vi "DDSBox.vi"() -> ()   [LabVIEW 2014]
uses:
  <vilib>/Utility/file.llb/Write To Spreadsheet File (DBL).vi
  <vilib>/Utility/file.llb/Read From Spreadsheet File (DBL).vi
panel:
  in  "Reset":bool=TRUE
  in  "stop":bool
  in  "Save":bool
  in  "Profile File":path=path "D:/app/DDS/DDSBox/DDSBox.csv"
  in  "Channel":u32(ring) items=["0", "1", "2", "3"]
  in  "Profiles":T1(array[cluster]) {"Phase (Pi)" min=0.0 max=2.0 format="%.2f"; "Amplitude" min=0.0 max=1.0 format="%.2f"; "Frequency (MHz)" min=0.0 max=500.0 format="%.6f"}
  in  "Port":refnum<visa-resource-name>="COM16"
  in  "Profile":u32(ring) items=["0", "1", "2", "3", "4", "5", "6", "7"]
  in  "Phase (Pi)":dbl min=0.0 max=2.0 format="%.2f"
  in  "Frequency (MHz)":dbl=200.0 min=0.0 max=500.0 format="%.6f"
  in  "Amplitude":dbl=1.0 min=0.0 max=1.0 format="%.2f"
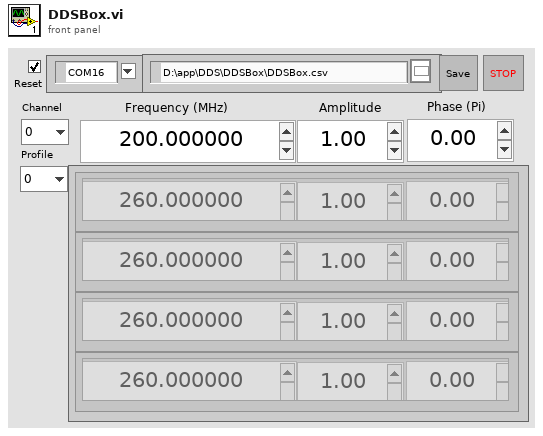
[diagram p1: front panel]
types:
  T1 = cluster{"Frequency (MHz) ":dbl, "Amplitude ":dbl, "Phase (Pi) ":dbl}[][]
  T2 = cluster{"Frequency (MHz) ":dbl, "Amplitude ":dbl, "Phase (Pi) ":dbl}
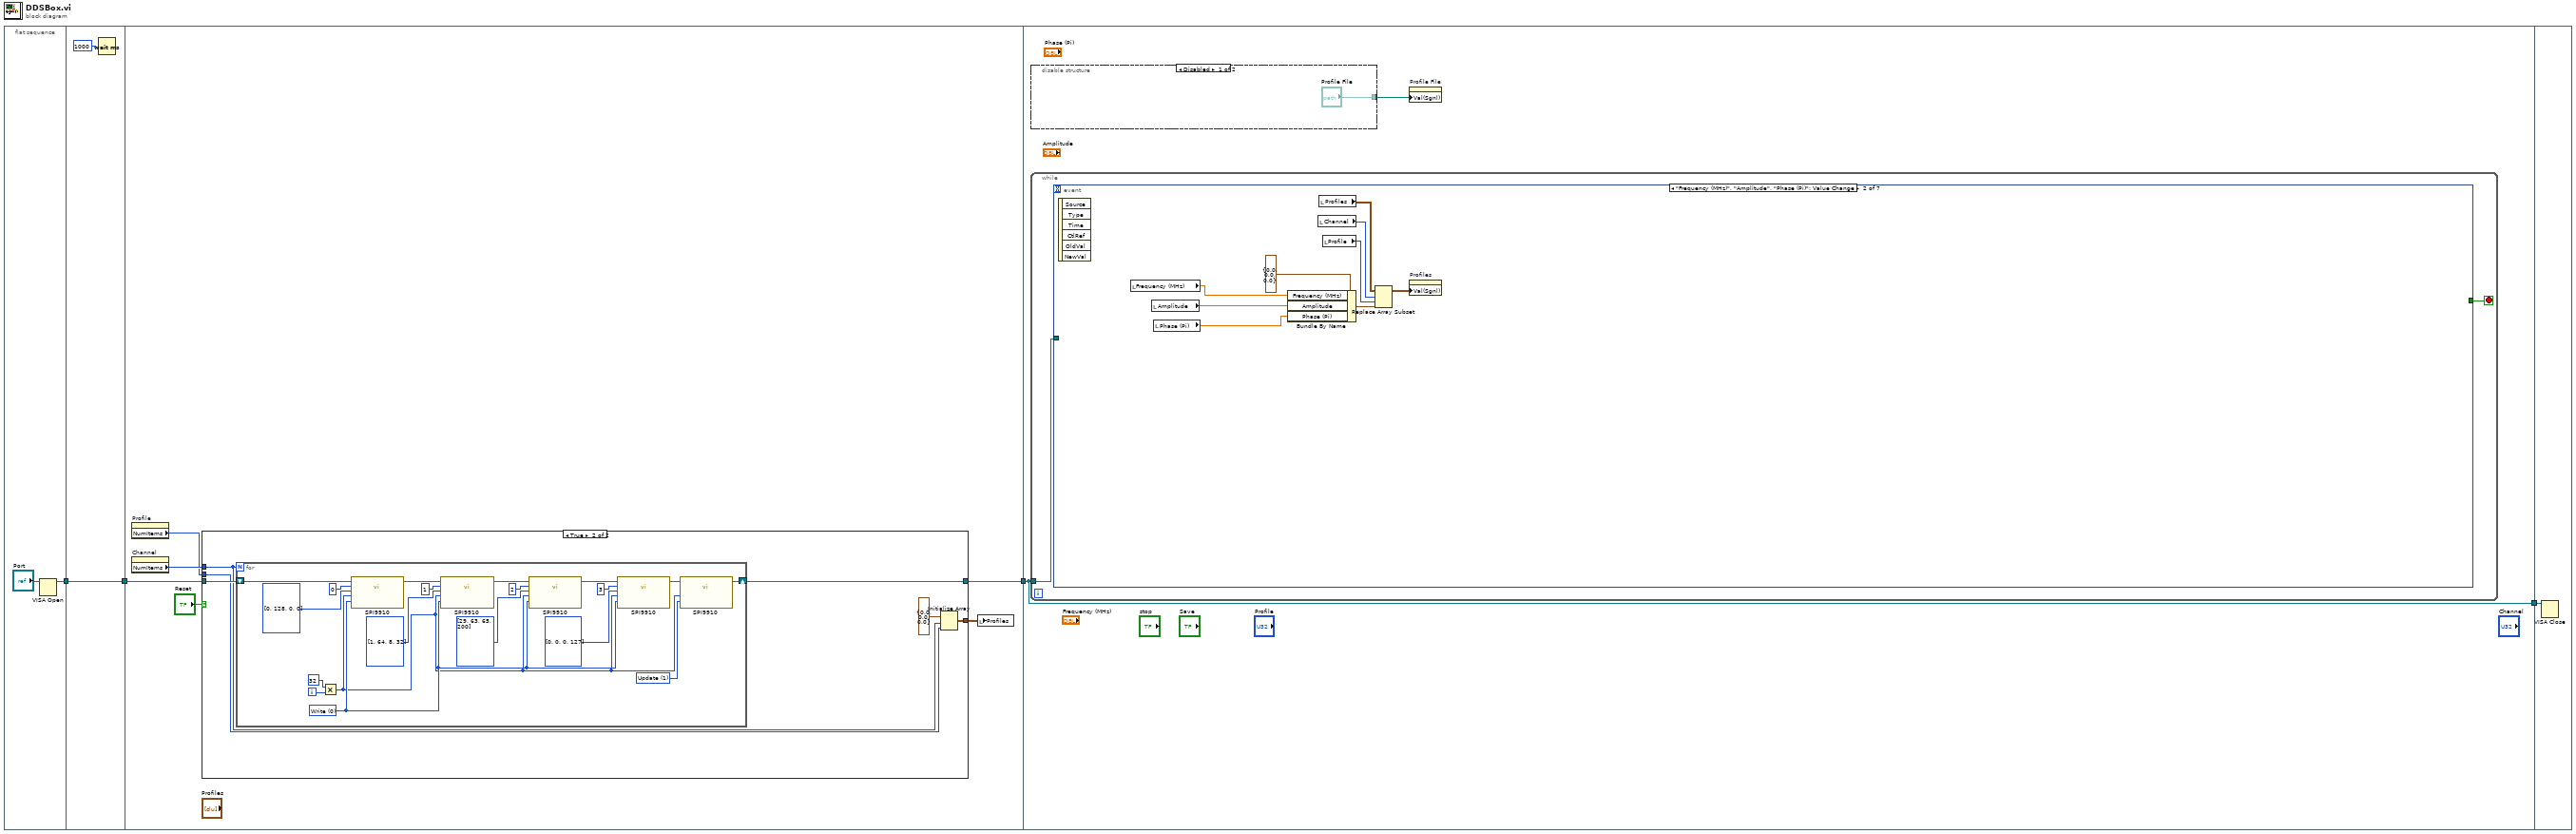
[diagram p0: block diagram]
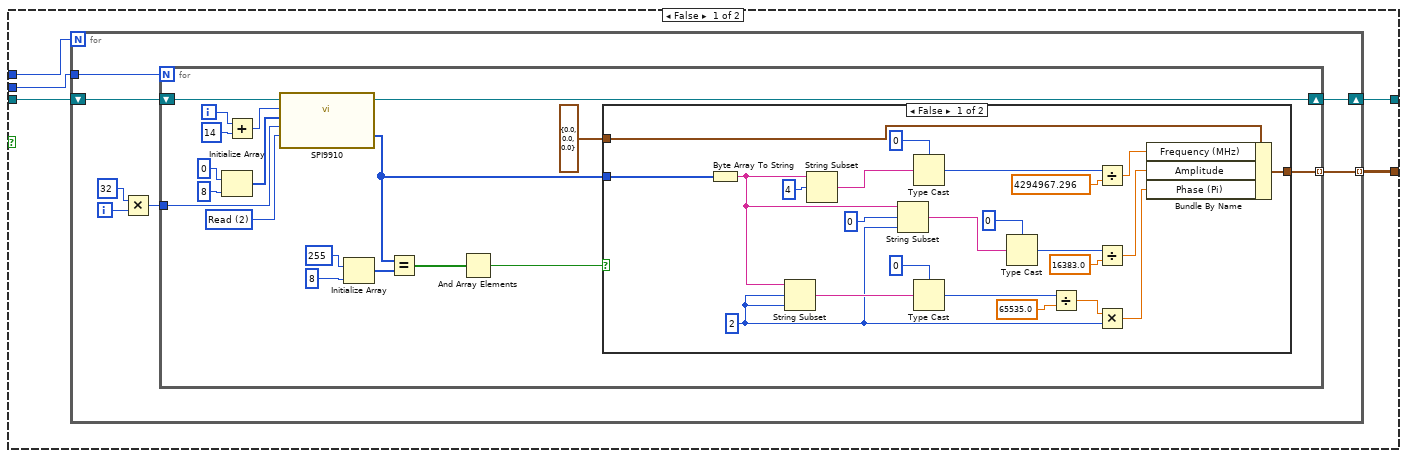
[diagram p2: hidden frame]
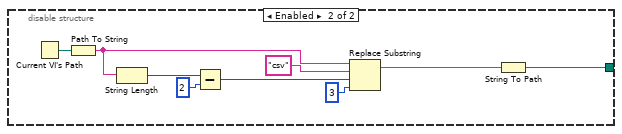
[diagram p4: hidden frame]
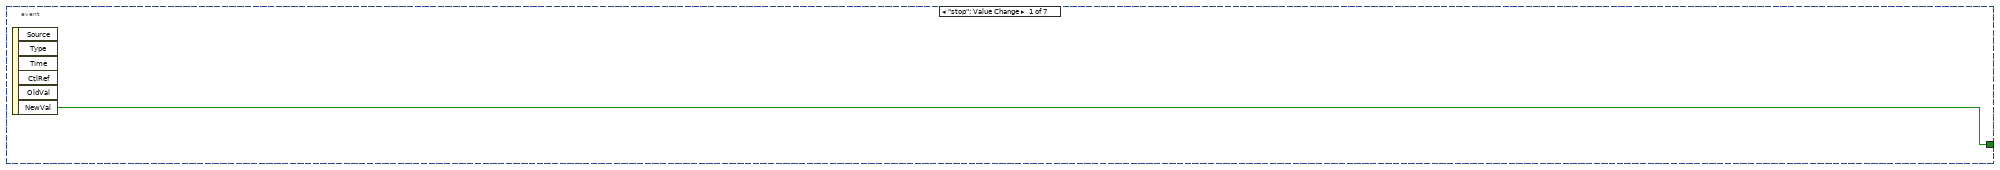
[diagram p5: hidden frame]
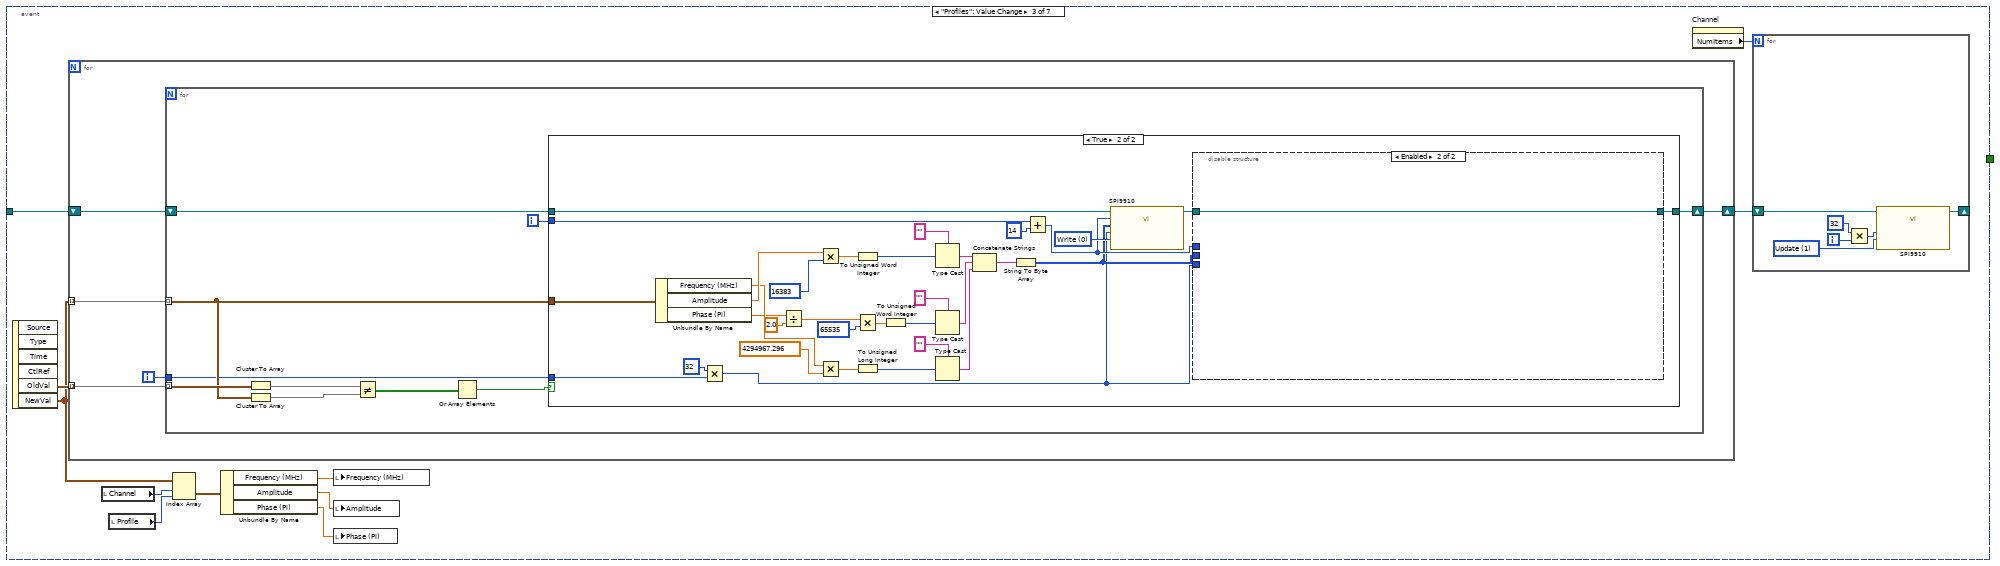
[diagram p6: hidden frame]
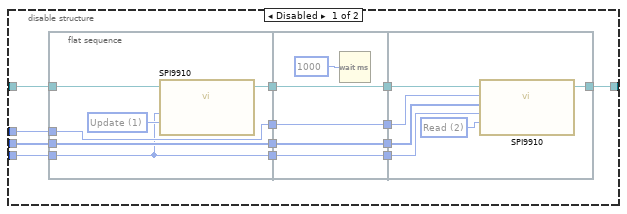
[diagram p8: hidden frame]
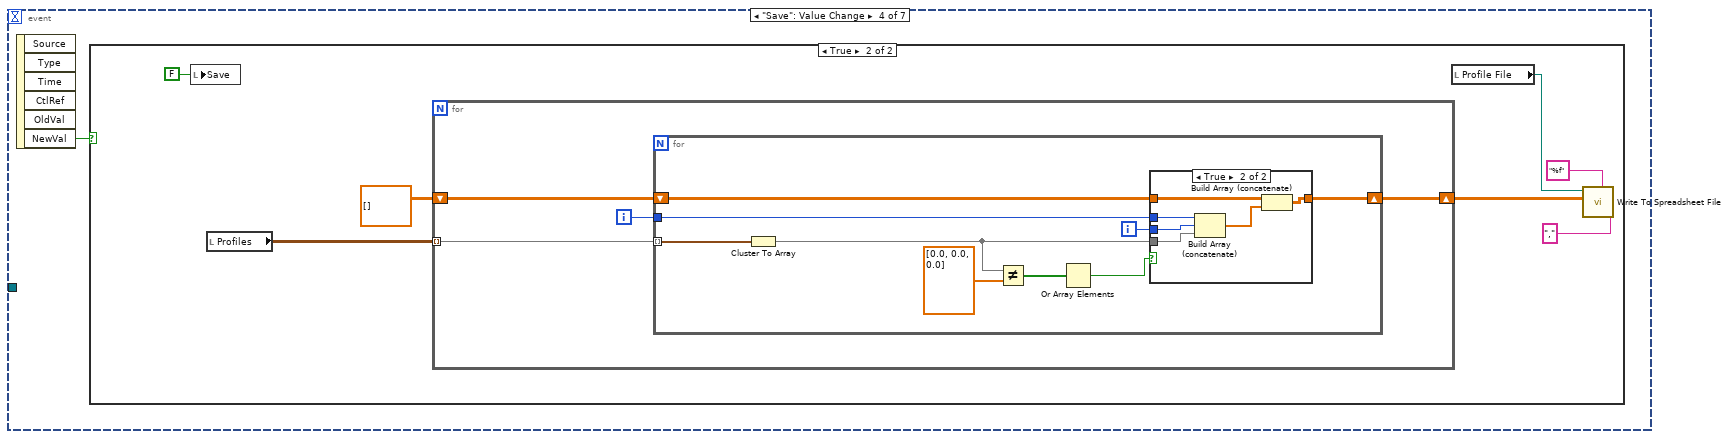
[diagram p9: hidden frame]
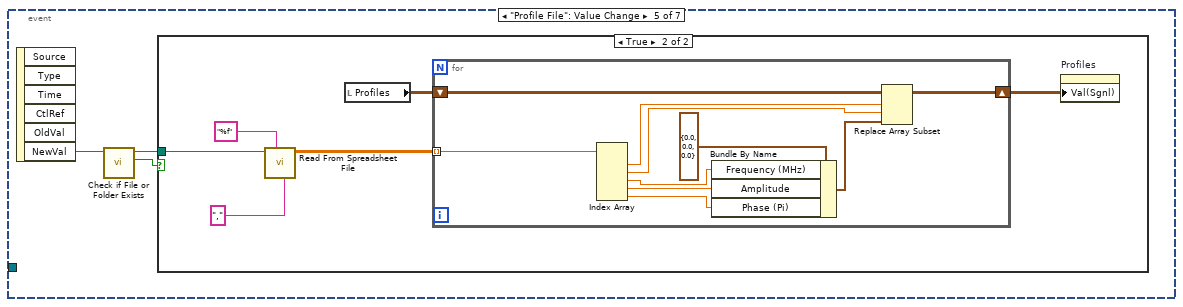
[diagram p12: hidden frame]
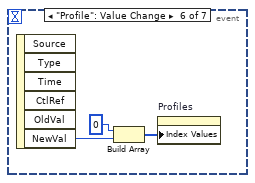
[diagram p14: hidden frame]
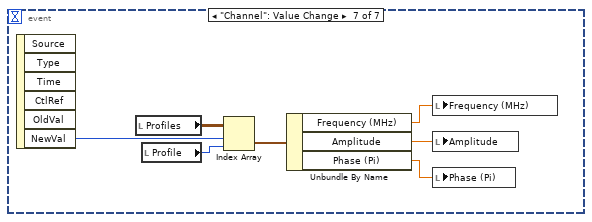
[diagram p15: hidden frame]
diagram:
  n1 = flat-sequence {
    tunnel: [w5] -> w2
    tunnel: w2 -> [w7]
    tunnel: [w7] -> w1
    tunnel: [w14] -> w3
    tunnel: w1 -> [w13]
    tunnel: w3 -> [w95]
    tunnel: [w95] -> w4
    tunnel: w4 -> [w272]
    frame #0 {
      n2 = VISA Open(VISA resource name="Port") -> (VISA resource name=w5:refnum<visa-resource-name>)  [unwired: 4 in, 1 out]
    }
    frame #1 {
      n3 = Wait (ms)(milliseconds to wait=u32 1000) -> ()  [unwired: 1 out]
    }
    frame #2 {
      n4 = property on="Profile" class="Ring (strict)"() -> ("NumItems"=w10:u32)  [unwired: 2 in, 2 out]
      n5 = property on="Channel" class="Ring (strict)"() -> ("NumItems"=w11:u32)  [unwired: 2 in, 2 out]
      n6 = case shown="True" "Reset" {
        tunnel: [w16 w74] -> w14
        tunnel: w13 -> [w17 w73]
        tunnel: [w15 w71] -> w9
        tunnel: w11 -> [w19 w70]
        tunnel: w10 -> [w18 w69]
        frame False {
          n7 = for {
            N: w19 -> [_]
            tunnel: w18 -> [w24]
            shift-right: [w21] -> w16
            shift-left: w17 -> [w23]
            tunnel: [w20] -> w15 mode=indexing
            i -> [w25]
            n8 = Multiply(x=32, y=w25) -> (x*y=w22:i32)
            n9 = for {
              N: w24 -> [_]
              shift-right: [w35] -> w21
              shift-left: w23 -> [w41]
              tunnel: w22 -> [w40]
              tunnel: [w34] -> w20 mode=indexing
              i -> [w43]
              w39 = u32 2 items=["Write", "Update", "Read"] ("Command")
              n10 = Initialize Array(u8 0 ("Byte"), 8 ("dimension size")) -> (w36:u8[])
              n11 = Add(x=w43, y=u8 14 ("Byte")) -> (x+y=w42:i32)
              n12 = call "SPI9910.vi"("Port In"=w41, "Register"=w42, "Input"=w36, "Offset"=w40, "Command"=w39) -> ("Port Out"=w35:refnum<visa-resource-name>, "Output"=w30:u8[])
              n13 = Initialize Array(u8 255 ("Byte"), 8 ("dimension size")) -> (w31:u8[])
              n14 = Equal?(x=w30, y=w31) -> (x = y?=w29:bool[])
              n15 = And Array Elements(Boolean array=w29) -> (logical AND=w28:bool)
              n16 = case shown="False" w28 {
                tunnel: [w47 w68] -> w34
                tunnel: w30 -> [w46 _]
                tunnel: T2 {"Frequency (MHz) "=0.0, "Amplitude "=0.0, "Phase (Pi) "=0.0} ("Profile") -> [w45 w68]
                frame False {
                  w57 = 2 ("length (rest)")
                  n17 = Byte Array To String(unsigned byte array=w46) -> (string=w55:string)
                  n18 = String Subset(string=w55, offset (0)=w57, length (rest)=w57) -> (substring=w61:string)
                  n19 = String Subset(string=w55, offset (0)=4) -> (substring=w53:string)  [unwired: 1 in]
                  n20 = String Subset(string=w55, offset (0)=0, length (rest)=w57) -> (substring=w66:string)
                  n21 = Type Cast(type=u32 0 ("Byte"), x=w53) -> (*(type *) &x=w52:u32)
                  n22 = Type Cast(type=u16 0 ("Byte"), x=w61) -> (*(type *) &x=w59:u16)
                  n23 = Type Cast(type=u16 0 ("Byte"), x=w66) -> (*(type *) &x=w63:u16)
                  n24 = Divide(x=w59, y=65535.0 ("Byte")) -> (x/y=w58:dbl)
                  n25 = Divide(x=w52, y=4294967.296 ("Byte")) -> (x/y=w50:dbl)
                  n26 = Divide(x=w63, y=16383.0 ("Byte")) -> (x/y=w49:dbl)
                  n27 = Multiply(x=w58, y=w57) -> (x*y=w48:dbl)
                  n28 = Bundle By Name(cluster=w45, "Frequency (MHz)"=w50, "Amplitude"=w49, "Phase (Pi)"=w48) -> (w47:T2)
                }
                frame True {
                }
              }
            }
          }
        }
        frame True {
          n29 = for {
            N: w70 -> [_]
            shift-right: [w77] -> w74
            shift-left: w73 -> [w93]
            i -> [w91]
            w76 = u32 1 items=["Write", "Update", "Read"] ("Command")
            w83 = u32 0 items=["Write", "Update", "Read"] ("Command")
            n30 = Multiply(x=32, y=w91) -> (x*y=w75:i32)
            n31 = call "SPI9910.vi"("Port In"=w93, "Register"=u8 0, "Input"=u8[] [0, 128, 0, 0], "Offset"=w75, "Command"=w83) -> ("Port Out"=w89:refnum<visa-resource-name>)  [unwired: 1 out]
            n32 = call "SPI9910.vi"("Port In"=w89, "Register"=u8 1, "Input"=u8[] [1, 64, 8, 32], "Offset"=w75, "Command"=w83) -> ("Port Out"=w88:refnum<visa-resource-name>)  [unwired: 1 out]
            n33 = call "SPI9910.vi"("Port In"=w88, "Register"=u8 2, "Input"=u8[] [29, 63, 65, 200], "Offset"=w75, "Command"=w83) -> ("Port Out"=w87:refnum<visa-resource-name>)  [unwired: 1 out]
            n34 = call "SPI9910.vi"("Port In"=w87, "Register"=u8 3, "Input"=u8[] [0, 0, 0, 127], "Offset"=w75, "Command"=w83) -> ("Port Out"=w78:refnum<visa-resource-name>)  [unwired: 1 out]
            n35 = call "SPI9910.vi"("Port In"=w78, "Offset"=w75, "Command"=w76) -> ("Port Out"=w77:refnum<visa-resource-name>)  [unwired: 2 in, 1 out]
          }
          n36 = Initialize Array(T2 {"Frequency (MHz) "=0.0, "Amplitude "=0.0, "Phase (Pi) "=0.0} ("Profile"), w70, w69) -> (w71:T1)
        }
      }
      n37 = local write "Profiles"(w9) -> ()
    }
    frame #3 {
      n38 = disable-structure shown="Disabled" {
        disable-tunnel: ["Profile File" w97] -> w94
        frame Disabled {
        }
        frame Enabled {
          n39 = Current VI's Path() -> (path=w105:path)
          n40 = Path To String(path=w105) -> (string=w103:string)
          n41 = String Length(string=w103) -> (length=w102:i32)
          n42 = Subtract(x=w102, y=2) -> (x-y=w100:i32)
          n43 = Replace Substring(2:3 ("length (len. of substring)"), 3:w100, 4:"csv" ("substring (\"\")"), 5:w103) -> (1:w98:string)  [unwired: 1 out]
          n44 = String To Path(string=w98) -> (path=w97:path)
        }
      }
      n45 = while {
        tunnel: w95 -> [w106]
        stop <- w107 stop-if-true
        n46 = event shown="[1] \"Frequency (MHz)\", \"Amplitude\", \"Phase (Pi)\": Value Change" {
          selector: _ -> [_ _ _ _ _ _ _]
          dyn-events: _ -> [_ _ _ _ _ _ _]
          timeout: _ -> [_ _ _ _ _ _ _]
          tunnel: [w108 _ _ _ _ _ _] -> w107
          tunnel: w106 -> [_ _ w128 _ _ _ _]
          event "stop": Value Change {
            n47 = event-data() -> ("NewVal"=w108:bool)  [unwired: 1 in, 5 out]
          }
          event "Frequency (MHz)", "Amplitude", "Phase (Pi)": Value Change {
            n48 = event-data() -> ()  [unwired: 1 in, 6 out]
            n49 = local read "Frequency (MHz)"() -> (w115:dbl)
            n50 = local read "Amplitude"() -> (w114:dbl)
            n51 = local read "Phase (Pi)"() -> (w113:dbl)
            n52 = Bundle By Name(cluster=T2 {"Frequency (MHz) "=0.0, "Amplitude "=0.0, "Phase (Pi) "=0.0} ("Profile"), "Frequency (MHz)"=w115, "Amplitude"=w114, "Phase (Pi)"=w113) -> (w112:T2)
            n53 = local read "Channel"() -> (w110:u32)
            n54 = local read "Profiles"() -> (w117:T1)
            n55 = local read "Profile"() -> (w111:u32)
            n56 = Replace Array Subset(array=w117, new element=w112, index (row)=w110, index (col)=w111) -> (w109:T1)
            n57 = property on="Profiles" class="Arr (strict)"("Val(Sgnl)"=w109) -> ()  [unwired: 2 in, 2 out]
          }
          event "Profiles": Value Change {
            n58 = event-data() -> ("OldVal"=w127:T1, "NewVal"=w124:T1)  [unwired: 1 in, 4 out]
            n59 = for {
              tunnel: w124 -> [w138] mode=indexing
              tunnel: w127 -> [w137] mode=indexing
              shift-right: [w135] -> w126
              shift-left: w128 -> [w139]
              i -> [w136]
              n60 = for {
                tunnel: w138 -> [w144] mode=indexing
                tunnel: w137 -> [w148] mode=indexing
                tunnel: w136 -> [w142]
                shift-right: [w140] -> w135
                shift-left: w139 -> [w149]
                i -> [w141]
                n61 = Cluster To Array(cluster=w148) -> (array=w147:dbl[])
                n62 = Cluster To Array(cluster=w144) -> (array=w146:dbl[])
                n63 = Not Equal?(x=w147, y=w146) -> (x != y?=w145:bool[])
                n64 = Or Array Elements(Boolean array=w145) -> (logical OR=w143:bool)
                n65 = case shown="True" w143 {
                  tunnel: w149 -> [w150 w183]
                  tunnel: w144 -> [_ w158]
                  tunnel: w142 -> [_ w152]
                  tunnel: w141 -> [_ w151]
                  tunnel: [w150 w153] -> w140
                  frame False {
                  }
                  frame True {
                    w182 = u32 0 items=["Write", "Update", "Read"] ("Command")
                    n66 = Unbundle By Name(w158) -> ("Frequency (MHz)"=w156:dbl, "Amplitude"=w157:dbl, "Phase (Pi)"=w155:dbl)
                    n67 = Multiply(x=u8 32, y=w152) -> (x*y=w159:i32)
                    n68 = Divide(x=w155, y=2.0) -> (x/y=w170:dbl)
                    n69 = Multiply(x=w157, y=u16 16383 ("Byte")) -> (x*y=w178:dbl)
                    n70 = Multiply(x=w156, y=4294967.296 ("Byte")) -> (x*y=w168:dbl)
                    n71 = To Unsigned Word Integer(number=w178) -> (unsigned 16bit integer=w177:u16)
                    n72 = Multiply(x=w170, y=u16 65535 ("Byte")) -> (x*y=w173:dbl)
                    n73 = To Unsigned Long Integer(number=w168) -> (unsigned 32bit integer=w166:u32)
                    n74 = To Unsigned Word Integer(number=w173) -> (unsigned 16bit integer=w174:u16)
                    n75 = Type Cast(type="", x=w177) -> (*(type *) &x=w165:string)
                    n76 = Type Cast(type="", x=w174) -> (*(type *) &x=w164:string)
                    n77 = Type Cast(type="", x=w166) -> (*(type *) &x=w163:string)
                    n78 = Concatenate Strings(w165, w164, w163) -> (w162:string)
                    n79 = String To Byte Array(string=w162) -> (unsigned byte array=w160:u8[])
                    n80 = Add(x=w151, y=u8 14 ("Byte")) -> (x+y=w161:i32)
                    n81 = call "SPI9910.vi"("Port In"=w183, "Register"=w161, "Input"=w160, "Offset"=w159, "Command"=w182) -> ("Port Out"=w154:refnum<visa-resource-name>)  [unwired: 1 out]
                    n82 = disable-structure shown="Enabled" {
                      disable-tunnel: w161 -> [w196 _]
                      disable-tunnel: w160 -> [w195 _]
                      disable-tunnel: w159 -> [w194 _]
                      disable-tunnel: w154 -> [w185 w214]
                      disable-tunnel: [w184 w214] -> w153
                      frame Disabled {
                        n83 = flat-sequence {
                          tunnel: w194 -> [w197]
                          tunnel: w195 -> [w201]
                          tunnel: w196 -> [w202]
                          tunnel: [w202] -> w189
                          tunnel: [w201] -> w188
                          tunnel: [w197] -> w187
                          tunnel: [w200] -> w186
                          tunnel: w185 -> [w199]
                          tunnel: [w204] -> w193
                          tunnel: [w207] -> w192
                          tunnel: [w206] -> w191
                          tunnel: [w205] -> w190
                          tunnel: w189 -> [w204]
                          tunnel: w188 -> [w207]
                          tunnel: w187 -> [w206]
                          tunnel: w186 -> [w205]
                          tunnel: w193 -> [w213]
                          tunnel: w192 -> [w212]
                          tunnel: w191 -> [w211]
                          tunnel: w190 -> [w209]
                          tunnel: [w208] -> w184
                          frame #0 {
                            w198 = u32 1 items=["Write", "Update", "Read"] ("Command")
                            n84 = call "SPI9910.vi"("Port In"=w199, "Offset"=w197, "Command"=w198) -> ("Port Out"=w200:refnum<visa-resource-name>)  [unwired: 2 in, 1 out]
                          }
                          frame #1 {
                            n85 = Wait (ms)(milliseconds to wait=u32 1000 ("millisecond timer value")) -> ()  [unwired: 1 out]
                          }
                          frame #2 {
                            w210 = u32 2 items=["Write", "Update", "Read"] ("Command")
                            n86 = call "SPI9910.vi"("Port In"=w209, "Register"=w213, "Input"=w212, "Offset"=w211, "Command"=w210) -> ("Port Out"=w208:refnum<visa-resource-name>)  [unwired: 1 out]
                          }
                        }
                      }
                      frame Enabled {
                      }
                    }
                  }
                }
              }
            }
            n87 = local read "Channel"() -> (w123:u32)
            n88 = local read "Profile"() -> (w122:u32)
            n89 = Index Array(array=w124, index (row)=w123, index (col)=w122) -> (element=w121:T2)
            n90 = Unbundle By Name(w121) -> ("Frequency (MHz)"=w120:dbl, "Amplitude"=w119:dbl, "Phase (Pi)"=w118:dbl)
            n91 = local write "Frequency (MHz)"(w120) -> ()
            n92 = local write "Amplitude"(w119) -> ()
            n93 = local write "Phase (Pi)"(w118) -> ()
            n94 = property on="Channel" class="Ring (strict)"() -> ("NumItems"=w125:u32)  [unwired: 2 in, 2 out]
            n95 = for {
              N: w125 -> [_]
              shift-right: [w129] -> _
              shift-left: w126 -> [w134]
              i -> [w131]
              w133 = u32 1 items=["Write", "Update", "Read"] ("Command")
              n96 = Multiply(x=u8 32, y=w131) -> (x*y=w130:i32)
              n97 = call "SPI9910.vi"("Port In"=w134, "Offset"=w130, "Command"=w133) -> ("Port Out"=w129:refnum<visa-resource-name>)  [unwired: 2 in, 1 out]
            }
          }
          event "Save": Value Change {
            n98 = event-data() -> ("NewVal"=w215:bool)  [unwired: 1 in, 5 out]
            n99 = case shown="True" w215 {
              frame False {
              }
              frame True {
                n100 = local write "Save"(FALSE) -> ()
                n101 = local read "Profiles"() -> (w222:T1)
                n102 = for {
                  tunnel: w222 -> [w226] mode=indexing
                  shift-right: [w224] -> w220
                  shift-left: dbl[][] [] -> [w225]
                  i -> [w223]
                  n103 = for {
                    tunnel: w226 -> [w235] mode=indexing
                    shift-right: [w230] -> w224
                    shift-left: w225 -> [w231]
                    tunnel: w223 -> [w228]
                    i -> [w227]
                    n104 = Cluster To Array(cluster=w235) -> (array=w229:dbl[])
                    n105 = Not Equal?(x=w229, y=dbl[] [0.0, 0.0, 0.0]) -> (x != y?=w233:bool[])
                    n106 = Or Array Elements(Boolean array=w233) -> (logical OR=w232:bool)
                    n107 = case shown="True" w232 {
                      tunnel: w231 -> [w236 w242]
                      tunnel: [w236 w241] -> w230
                      tunnel: w229 -> [_ w240]
                      tunnel: w228 -> [_ w239]
                      tunnel: w227 -> [_ w238]
                      frame False {
                      }
                      frame True {
                        n108 = Build Array (concatenate)(w239, w238, w240) -> (w237:dbl[])
                        n109 = Build Array (concatenate)(w242, w237) -> (w241:dbl[][])
                      }
                    }
                  }
                }
                n110 = local read "Profile File"() -> (w218:path)
                n111 = call-poly <vilib>:"Write To Spreadsheet File.vi"("delimiter (\\t)"="," ("delimiter (\\t)"), "format (%.3f)"="%f", "2D data"=w220, "file path (dialog if empty)"=w218) -> ()  [unwired: 4 in, 1 out]
              }
            }
          }
          event "Profile File": Value Change {
            n112 = event-data() -> ("NewVal"=w245:path)  [unwired: 1 in, 5 out]
            n113 = call <vilib>:"Check if File or Folder Exists.vi"("path"=w245) -> ("file or folder exists?"=w244:bool, "dup path"=w243:path)  [unwired: 8 in, 1 out]
            n114 = case shown="True" w244 {
              tunnel: w243 -> [_ w251]
              frame False {
              }
              frame True {
                n115 = call-poly <vilib>:"Read From Spreadsheet File.vi"("delimiter (\\t)"="," ("delimiter (\\t)"), "format (%.3f)"="%f", "file path (dialog if empty)"=w251) -> ("all rows"=w249:dbl[][])  [unwired: 4 in, 4 out]
                n116 = local read "Profiles"() -> (w248:T1)
                n117 = for {
                  tunnel: w249 -> [w261] mode=indexing
                  shift-right: [w252] -> w247
                  shift-left: w248 -> [w253]
                  n118 = Index Array(array=w261) -> (element #1=w260:dbl, element #2=w259:dbl, element #3=w257:dbl, element #4=w256:dbl, element #5=w255:dbl)  [unwired: 5 in]
                  n119 = Bundle By Name(cluster=T2 {"Frequency (MHz) "=0.0, "Amplitude "=0.0, "Phase (Pi) "=0.0} ("Profile"), "Frequency (MHz)"=w257, "Amplitude"=w256, "Phase (Pi)"=w255) -> (w254:T2)
                  n120 = Replace Array Subset(array=w253, new element=w254, index (row)=w260, index (col)=w259) -> (w252:T1)
                }
                n121 = property on="Profiles" class="Arr (strict)"("Val(Sgnl)"=w247) -> ()  [unwired: 2 in, 2 out]
              }
            }
          }
          event "Profile": Value Change {
            n122 = event-data() -> ("NewVal"=w262:u32)  [unwired: 1 in, 5 out]
            n123 = Build Array(u32 0 ("element"), w262) -> (w264:u32[])
            n124 = property on="Profiles" class="Arr (strict)"("Index Values"=w264) -> ()  [unwired: 2 in, 2 out]
          }
          event "Channel": Value Change {
            n125 = event-data() -> ("NewVal"=w266:u32)  [unwired: 1 in, 5 out]
            n126 = local read "Profiles"() -> (w271:T1)
            n127 = local read "Profile"() -> (w265:u32)
            n128 = Index Array(array=w271, index (row)=w266, index (col)=w265) -> (element=w270:T2)
            n129 = Unbundle By Name(w270) -> ("Frequency (MHz)"=w269:dbl, "Amplitude"=w268:dbl, "Phase (Pi)"=w267:dbl)
            n130 = local write "Frequency (MHz)"(w269) -> ()
            n131 = local write "Amplitude"(w268) -> ()
            n132 = local write "Phase (Pi)"(w267) -> ()
          }
        }
      }
      n133 = property on="Profile File" class="Path"("Val(Sgnl)"=w94) -> ()  [unwired: 2 in, 2 out]
    }
    frame #4 {
      n134 = VISA Close(VISA resource name=w272) -> ()  [unwired: 1 in, 1 out]
    }
  }
